vi "Msg.vi"(7 "Actor in":refnum<class "Actor.lvclass">, 11 "Queue Create Msg in":refnum<class "Queue Create Msg.lvclass">) -> (5 "Actor out":refnum<class "Actor.lvclass">)   [LabVIEW 2021, in "jettl.lvlib" / "Queue Create.lvlib" / "Queue Create Msg.lvclass"]
uses:
  Queue Create Msg.lvclass
  Actor/Actor.lvclass
  Queue Create/Queue Create.lvclass
  Queue Create Msg.lvclass/Queue Create Msg.ctl
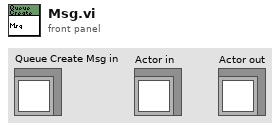
[diagram p1: front panel]
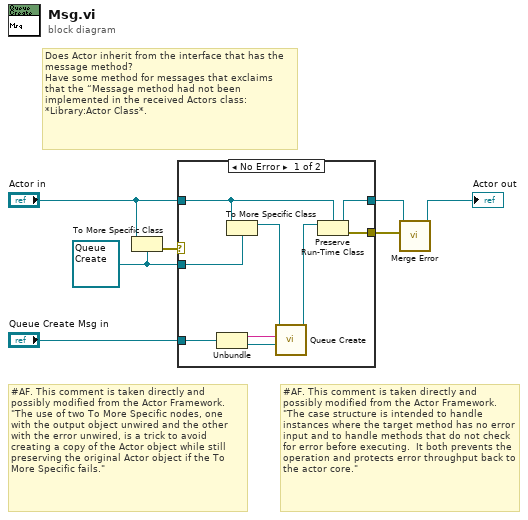
[diagram p0: block diagram]
diagram:
  w6 = refnum<class "Queue Create.lvclass"> refnum ("Create.lvlib:Create.lvclass")
  # "#AF. This comment is taken directly and possibly modified from the Actor Framework.\n\"The use of two To More Specific nodes, one with the output object unwired and the other with the error unwired, is a trick to avoid creating a copy of the Actor object while still preserving the original Actor object if the To More Specific fails.\""
  # "#AF. This comment is taken directly and possibly modified from the Actor Framework.\n\"The case structure is intended to handle instances where the target method has no error input and to handle methods that do not check for error before executing.  It both prevents the operation and protects error throughput back to the actor core.\""
  # "Does Actor inherit from the interface that has the message method?\nHave some method for messages that exclaims that the “Message method had not been implemented in the received Actors class:\n*Library:Actor Class*."
  n1 = To More Specific Class(target class=w6, reference="Actor in") -> (error out=w7:errorcluster)  [unwired: 1 in, 1 out]
  n2 = case shown="No Error" w7 {
    selector: w7 -> [_ w17]
    tunnel: [w9 w18] -> w3
    tunnel: "Actor in" -> [w11 w18]
    tunnel: w6 -> [w15 _]
    tunnel: "Queue Create Msg in" -> [w14 _]
    tunnel: [w8 w17] -> w4
    frame No Error {
      n3 = Unbundle(w14) -> (w13:string, w12:refnum<class "Queue Actor.lvclass">)
      n4 = To More Specific Class(target class=w15, reference=w11) -> (specific class reference=w16:refnum<class "Queue Create.lvclass">)  [unwired: 1 in, 1 out]
      n5 = call-dynamic "Queue Create.vi"("Queue Actor"=w12, "Alias"=w13, "Queue Create in"=w16) -> ("Queue Create out"=w10:refnum<class "Queue Create.lvclass">)  [unwired: 8 in]
      n6 = Preserve Run-Time Class(object in=w10, 2:w11) -> (object out=w9:refnum<class "Actor.lvclass">, error out=w8:errorcluster)  [unwired: 1 in]
    }
    frame Error {
    }
  }
  n7 = call-dynamic "Merge Error.vi"("Error"=w4, "Set Error in"=w3) -> ("Set Error out"=→"Actor out":refnum<class "Actor.lvclass">)  [unwired: 9 in]
